vi "Collect Result.vi"(10 "Results":T1[](array[typedef]), 11 "Report Generator In":refnum<class "Result Collector.lvclass">) -> (3 "Report Generator Out":refnum<class "Result Collector.lvclass">)   [LabVIEW 2020, in "Result Collector.lvclass"]
uses:
  Result Collector.lvclass
  Rewrite Project/Result/Result.ctl
  Rewrite Project/Result/Status.ctl
  Rewrite Project/Result/Type.ctl
  Result Types/Case Result/Test Case Result.ctl
  Result Types/Method Result/Method Result.ctl
  Result Types/Assertion Result/Assertion Result.ctl
  Result Types/Assertion Result/Public/TypeDefs/Assertion Type.ctl
  Result Collector.lvclass/Result Collector.ctl
  Result Types/Suite Results/Test Suite Result.ctl
  Result Types/Assertion Result/Assertion Result.lvlib
  Result Types/Method Result/Method Result.lvlib
  Rewrite Project/Result/Result.lvlib
  Result Types/Case Result/Test Case Result.lvlib
  Result Types/Suite Results/Test Suite Result.lvlib
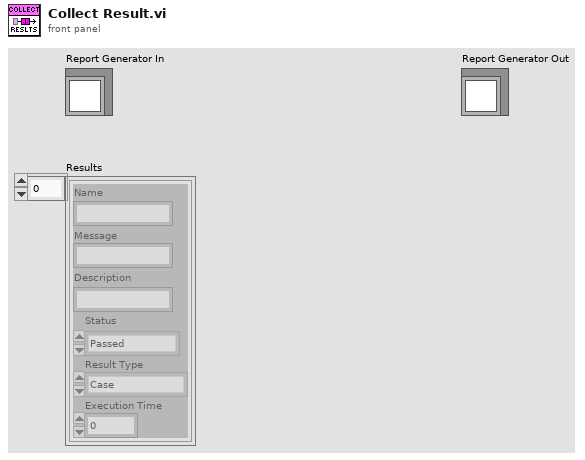
[diagram p1: front panel]
types:
  T1 = typedef "Result.lvlib/Result.ctl" = cluster{"Name":string, "Message":string, "Description":string, "Status":T2, "Result Type":T3, "Execution Time":dbl}
  T2 = typedef "Result.lvlib/Status.ctl" = enum16{"", "Passed", "Failed", "Error", "Skipped", "Setup Error", "Broken", "Teardown Error"}
  T3 = typedef "Result.lvlib/Type.ctl" = enum16{"Method", "Case", "Suite", "Pass", "Fail", "Skip", "Pass if", "Fail if", "Pass if Error", "Fail if Error", "Pass if Equal", "Fail if Equal"}
  T4 = typedef "Test Case Result.lvlib/Test Case Result.ctl" = map{string, T5}
  T5 = typedef "Method Result.lvlib/Method Result.ctl" = cluster{"Test Case":string, "Test Method Name":string, "Status":T2, "Assertion Results":T6[], "Execution time":dbl, "Result String":string}
  T6 = typedef "Assertion Result.lvlib/Assertion Result.ctl" = cluster{"Status":T2, "Message":string, "Description":string, "Assertion Type":T7}
  T7 = typedef "Result.lvlib/Assertion Type.ctl" = enum16{"None", "Pass", "Fail", "Skip", "Pass if Equal", "Fail if Equal", "Pass if Error", "Fail if Error", "Pass if", "Fail if"}
  T8 = typedef "Test Suite Result.lvlib/Test Suite Result.ctl" = cluster{"Test Suite ID":string, "Name":string, "Hostname":string, "Status":T2, "Execution time":dbl, "Start Time":timestamp, "Case Results":T4[]}
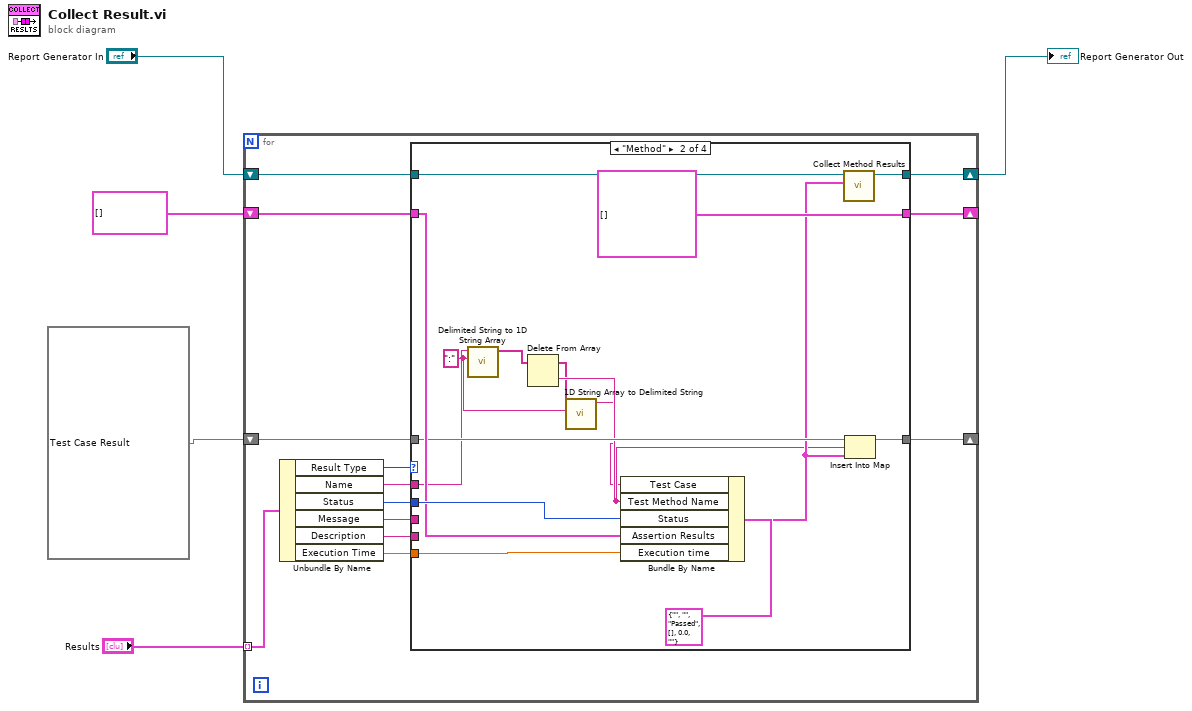
[diagram p0: block diagram]
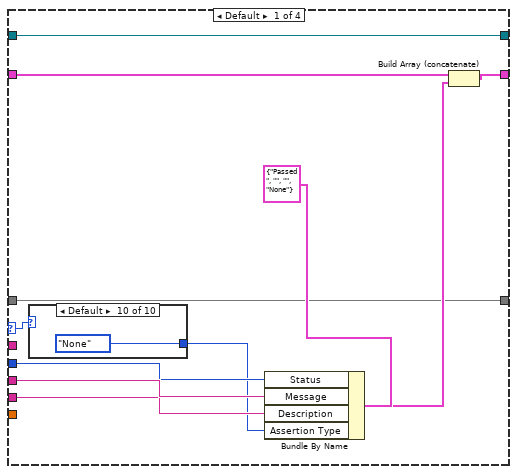
[diagram p2: hidden frame]
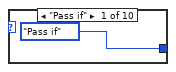
[diagram p3: hidden frame]
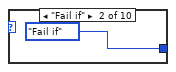
[diagram p4: hidden frame]
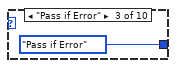
[diagram p5: hidden frame]
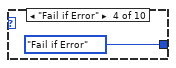
[diagram p6: hidden frame]
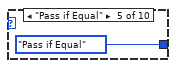
[diagram p7: hidden frame]
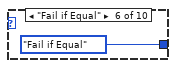
[diagram p8: hidden frame]
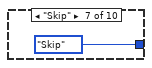
[diagram p9: hidden frame]
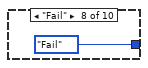
[diagram p10: hidden frame]
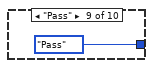
[diagram p11: hidden frame]
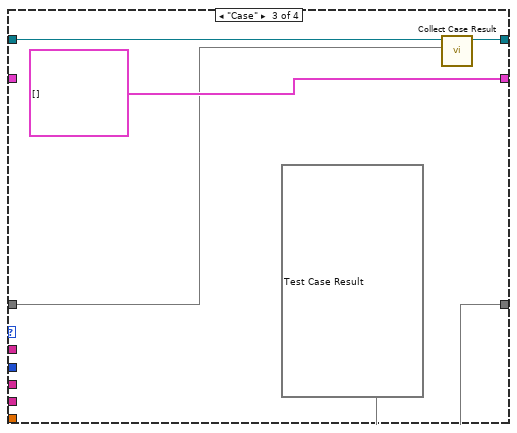
[diagram p12: hidden frame]
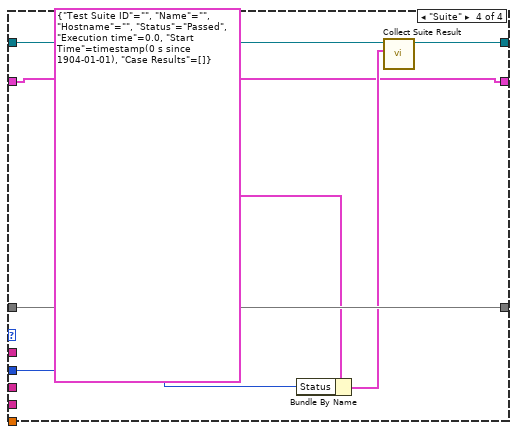
[diagram p13: hidden frame]
diagram:
  n1 = for {
    shift-right: [w17] -> w4
    shift-left: "Report Generator In" -> [w18]
    tunnel: "Results" -> [w15] mode=indexing
    shift-right: [w14] -> _
    shift-left: T6[] [] ("Assertion Results") -> [w11]
    shift-right: [w6] -> _
    shift-left: T4 {} ("Test Case Result") -> [w7]
    n2 = Unbundle By Name(w15) -> ("Result Type"=w16:T3, "Name"=w13:string, "Status"=w12:T2, "Message"=w10:string, "Description"=w9:string, "Execution Time"=w8:dbl)
    n3 = case shown="\"Method\"" w16 {
      selector: w16 -> [w19 _ _ _]
      tunnel: w18 -> [w28 w55 w60 w66]
      tunnel: [w28 w54 w59 w65] -> w17
      tunnel: w11 -> [w29 w51 _ w61]
      tunnel: [w27 T6[] [] ("Assertion Results") T6[] [] ("Assertion Results") w61] -> w14
      tunnel: w13 -> [_ w45 _ _]
      tunnel: w12 -> [w22 w52 _ w62]
      tunnel: w10 -> [w24 _ _ _]
      tunnel: w9 -> [w23 _ _ _]
      tunnel: w8 -> [_ w49 _ _]
      tunnel: w7 -> [w21 w48 w57 w67]
      tunnel: [w21 w47 T4 {} ("Test Case Result") w67] -> w6
      frame Default {
        n4 = case shown="Default" w19 {
          tunnel: [Assertion_Type."Pass if" ("Assertion Type") Assertion_Type."Fail if" ("Assertion Type") Assertion_Type."Pass if Error" ("Assertion Type") Assertion_Type."Fail if Error" ("Assertion Type") Assertion_Type."Pass if Equal" ("Assertion Type") Assertion_Type."Fail if Equal" ("Assertion Type") Assertion_Type."Skip" ("Assertion Type") Assertion_Type."Fail" ("Assertion Type") Assertion_Type."Pass" ("Assertion Type") Assertion_Type."None" ("Assertion Type")] -> w20
          frame "Pass if" {
          }
          frame "Fail if" {
          }
          frame "Pass if Error" {
          }
          frame "Fail if Error" {
          }
          frame "Pass if Equal" {
          }
          frame "Fail if Equal" {
          }
          frame "Skip" {
          }
          frame "Fail" {
          }
          frame "Pass" {
          }
          frame Default {
          }
        }
        n5 = Bundle By Name(cluster=T6 {"Status"=enum."Passed", "Message"="", "Description"="", "Assertion Type"=enum."None"} ("element"), "Status"=w22, "Message"=w24, "Description"=w23, "Assertion Type"=w20) -> (w25:T6)
        n6 = Build Array (concatenate)(w29, w25) -> (w27:T6[])
      }
      frame "Method" {
        w42 = ":" ("delimiter")
        n7 = call <vilib>:"Delimited String to 1D String Array.vi"("delimiter"=w42, "delimited string"=w45) -> ("string array"=w44:string[])  [unwired: 9 in]
        n8 = Delete From Array(array=w44) -> (deleted portion=w43:string, array with subset deleted=w41:string[])  [unwired: 2 in]
        n9 = call <vilib>:"1D String Array to Delimited String.vi"("delimiter"=w42, "string array"=w41) -> ("delimited string"=w40:string)  [unwired: 9 in]
        n10 = Bundle By Name(cluster=T5 {"Test Case"="", "Test Method Name"="", "Status"=enum."Passed", "Assertion Results"=[], "Execution time"=0.0, "Result String"=""} ("Test Method Result"), "Test Case"=w40, "Test Method Name"=w43, "Status"=w52, "Assertion Results"=w51, "Execution time"=w49) -> (w46:T5)
        n11 = call "Collect Method Results.vi"("Test Method Result"=w46, "Report Generator In"=w55) -> ("Report Generator Out"=w54:refnum<class "Result Collector.lvclass">)  [unwired: 9 in]
        n12 = Insert Into Map(map in=w48, key=w43, value=w46) -> (map out=w47:T4)  [unwired: 2 out]
      }
      frame "Case" {
        n13 = call "Collect Case Result.vi"("Test Case Result"=w57, "Report Generator In"=w60) -> ("Report Generator Out"=w59:refnum<class "Result Collector.lvclass">)  [unwired: 9 in]
      }
      frame "Suite" {
        n14 = Bundle By Name(cluster=T8 {"Test Suite ID"="", "Name"="", "Hostname"="", "Status"=enum."Passed", "Execution time"=0.0, "Start Time"=timestamp(0 s since 1904-01-01), "Case Results"=[]} ("Test Suite Result"), "Status"=w62) -> (w63:T8)
        n15 = call "Collect Suite Result.vi"("Test Suite Result"=w63, "Report Generator In"=w66) -> ("Report Generator Out"=w65:refnum<class "Result Collector.lvclass">)  [unwired: 8 in, 1 out]
      }
    }
  }
  "Report Generator Out" <- w4
